vi "TAT_Manual.vi"(8 "error In":errorcluster) -> (0 "error out":errorcluster)   [LabVIEW 2017]
uses:
  <vilib>/addons/database/Connection.llb/Conn ObjectReference.ctl
  <vilib>/Utility/error.llb/DialogType.ctl
  Controls/Ass. Loop Control.ctl
  b57a9467-0384-43c0-b8a9-3ecd2744b4aa.vi
  <vilib>/Instr/_visa.llb/VISA Configure Serial Port (Instr).vi
  <vilib>/Utility/config.llb/Read Key (I32).vi
  <vilib>/addons/database/NI_Database_API.lvlib
  <vilib>/Utility/config.llb/NI_LVConfig.lvlib
  def1aff2-28af-4330-adfa-ddbbffd99805.vi
panel:
  in  "Varient Change":bool
  out "12 4":bool
  out "12 2":bool
  out "12":bool
  in  "temp":refnum<visa-resource-name>
  out "array":string[](array[string])
  out "LEAK UNIT RESULT 2":bool caption="LEAK RESULT:-"
  out "LEAK ACTUAL VALUE 2":string
  out "LEAK MAX 2":string
  out "LEAK MIN 2":string
  out "LEAK UNIT RESULT":bool caption="LEAK RESULT:-"
  out "LEAK ACTUAL VALUE":string
  out "LEAK MAX":string
  out "LEAK MIN":string
  out "PREVIOUS BARCODE":string[](array[string])
  out "scanned":string
  out "Scanned Qyt":string
  out "PROJECT :-":string
  out "PACKAGE Qty":string
  out "TORISHI CODE:-":string
  out "PART No.:-":string
  in  "Stop":bool
  out "BARCODE STATION 2":string caption="BARCODE:-"
  out "RESULT STATION 1":bool caption="FINAL RESULT:-"
  out "USER:-":string
  out "PART NAME :-":string
  in  "ASS-Alarms":bool
  out "CYCLE STATUS STATION 1":string caption="CYCLE STATUS:-"
  out "DATE/TIME":string
  # "KAPSE SONS ROBOTICS\n& AUTOMATION"
  # "PROGRAM SELECTION"
  # "PREVIOUS BARCODE"
  # "Nm"
  # "POKA-YOKE STATUS"
  # "LEAK TESTING PARAMETER"
  # "MIN"
  # "MAX"
  # "ACTUAL VALUE"
  # "RESULT"
  # "LEAK UNIT"
  # "LEAK PRESSURE"
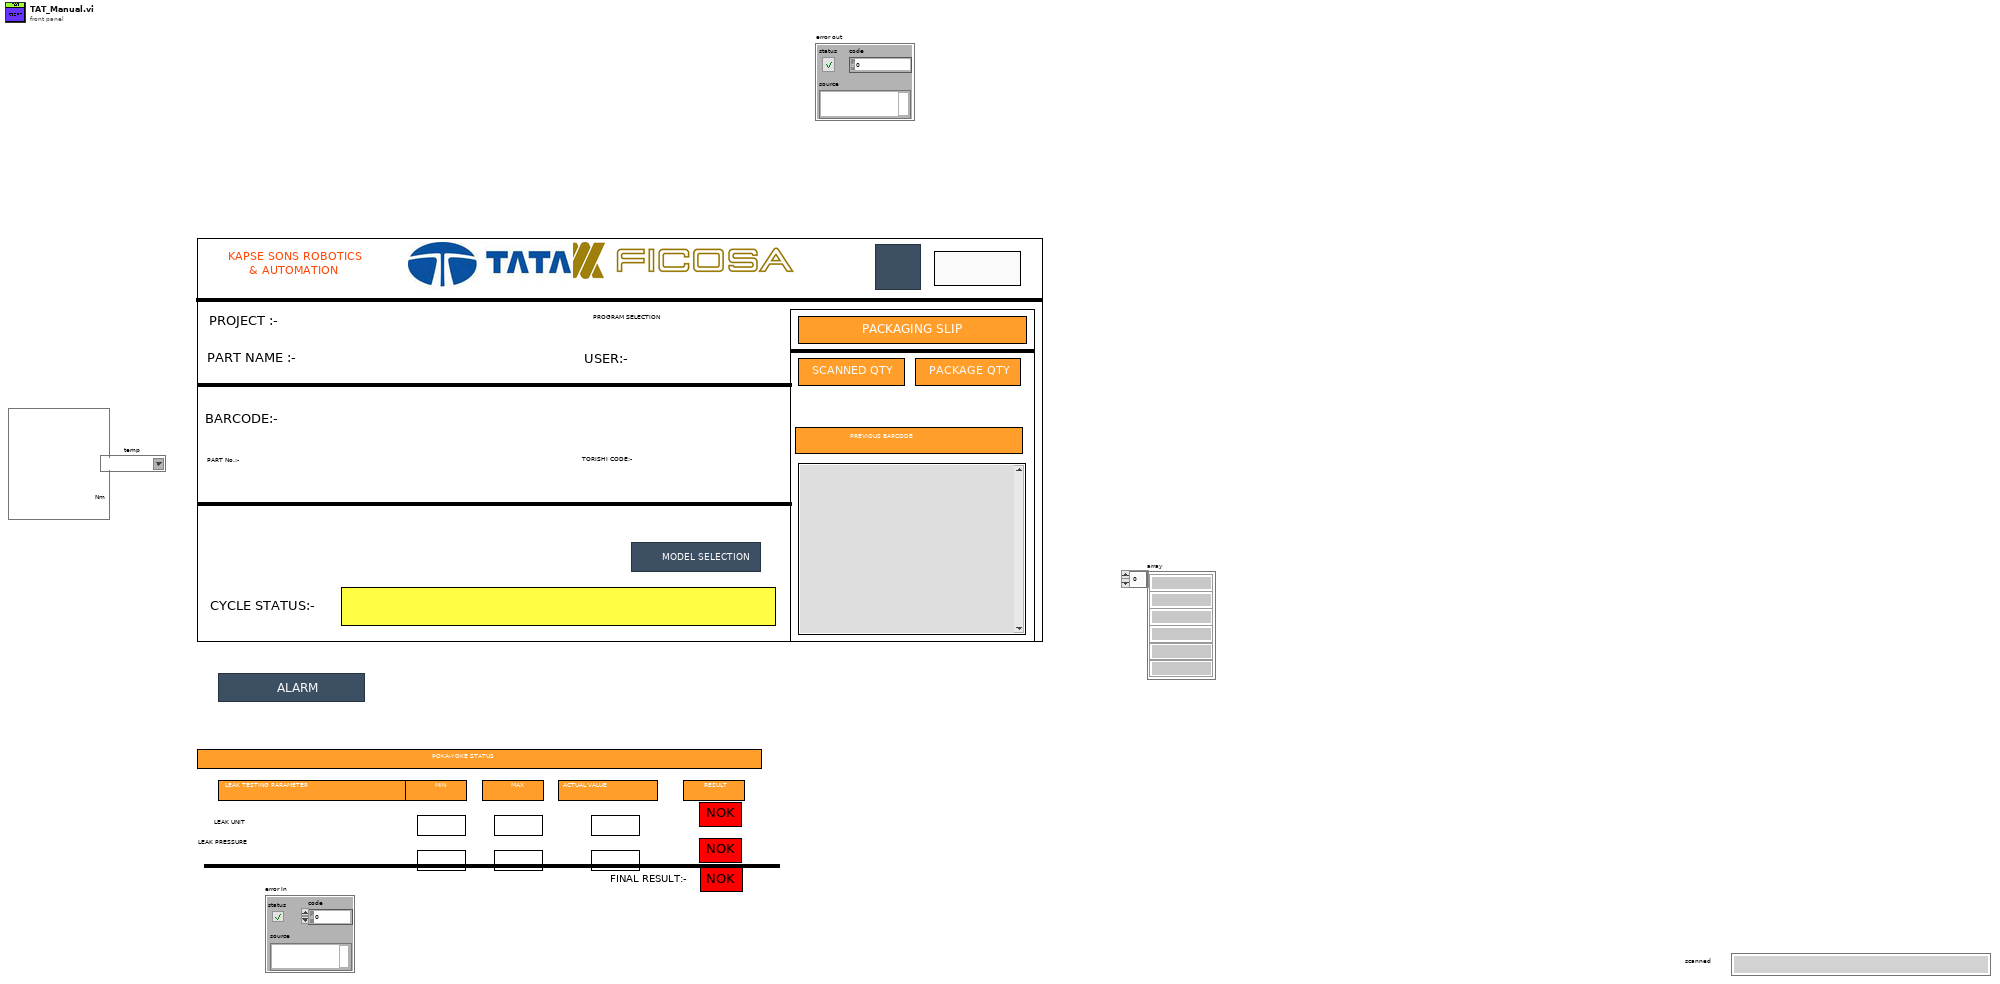
[diagram p1: front panel]
types:
  T1 = typedef "Ass. Loop Control.ctl" = enum16{"Int2", "Package_Qty_Count", "GENERATE_QR_PRNT", "Cluster_update", "Waiting_for_scan", "barcode CHECK", "Int", "SaveReport ", "Barcode Print", "Start Cycle", "Wait", "Cycle End", "Stop"}
  T2 = typedef "DialogType.ctl" = u16
  T3 = typedef "NI_Database_API.lvlib/Conn ObjectReference.ctl" = refnum<k1>
  T4 = cluster{"Varient number":u16, "Part name":string, "Barcode":string, "connection reference":T3, "Batch_Size":u16, "PART_NO":string, "TORISHI_CODE":string, "scanner com":refnum<visa-resource-name>, "Part Name List":string[], "Varient path":path, "Current Varient path":path, "Communication path":path, "PRN path":path, "printer":refnum<k5>, "Data_log_Path":path, "PREVIOUS Code":string[], "printer ip add":string}
  T5 = enum32{"invalid app kind", "Development System", "Run Time System", "Student Edition", "Embedded LabVIEW", "Evaluation", "Custom"}
  T6 = typedef "NI_LVConfig.lvlib/Config Data RefNum.ctl" = refnum<k1>
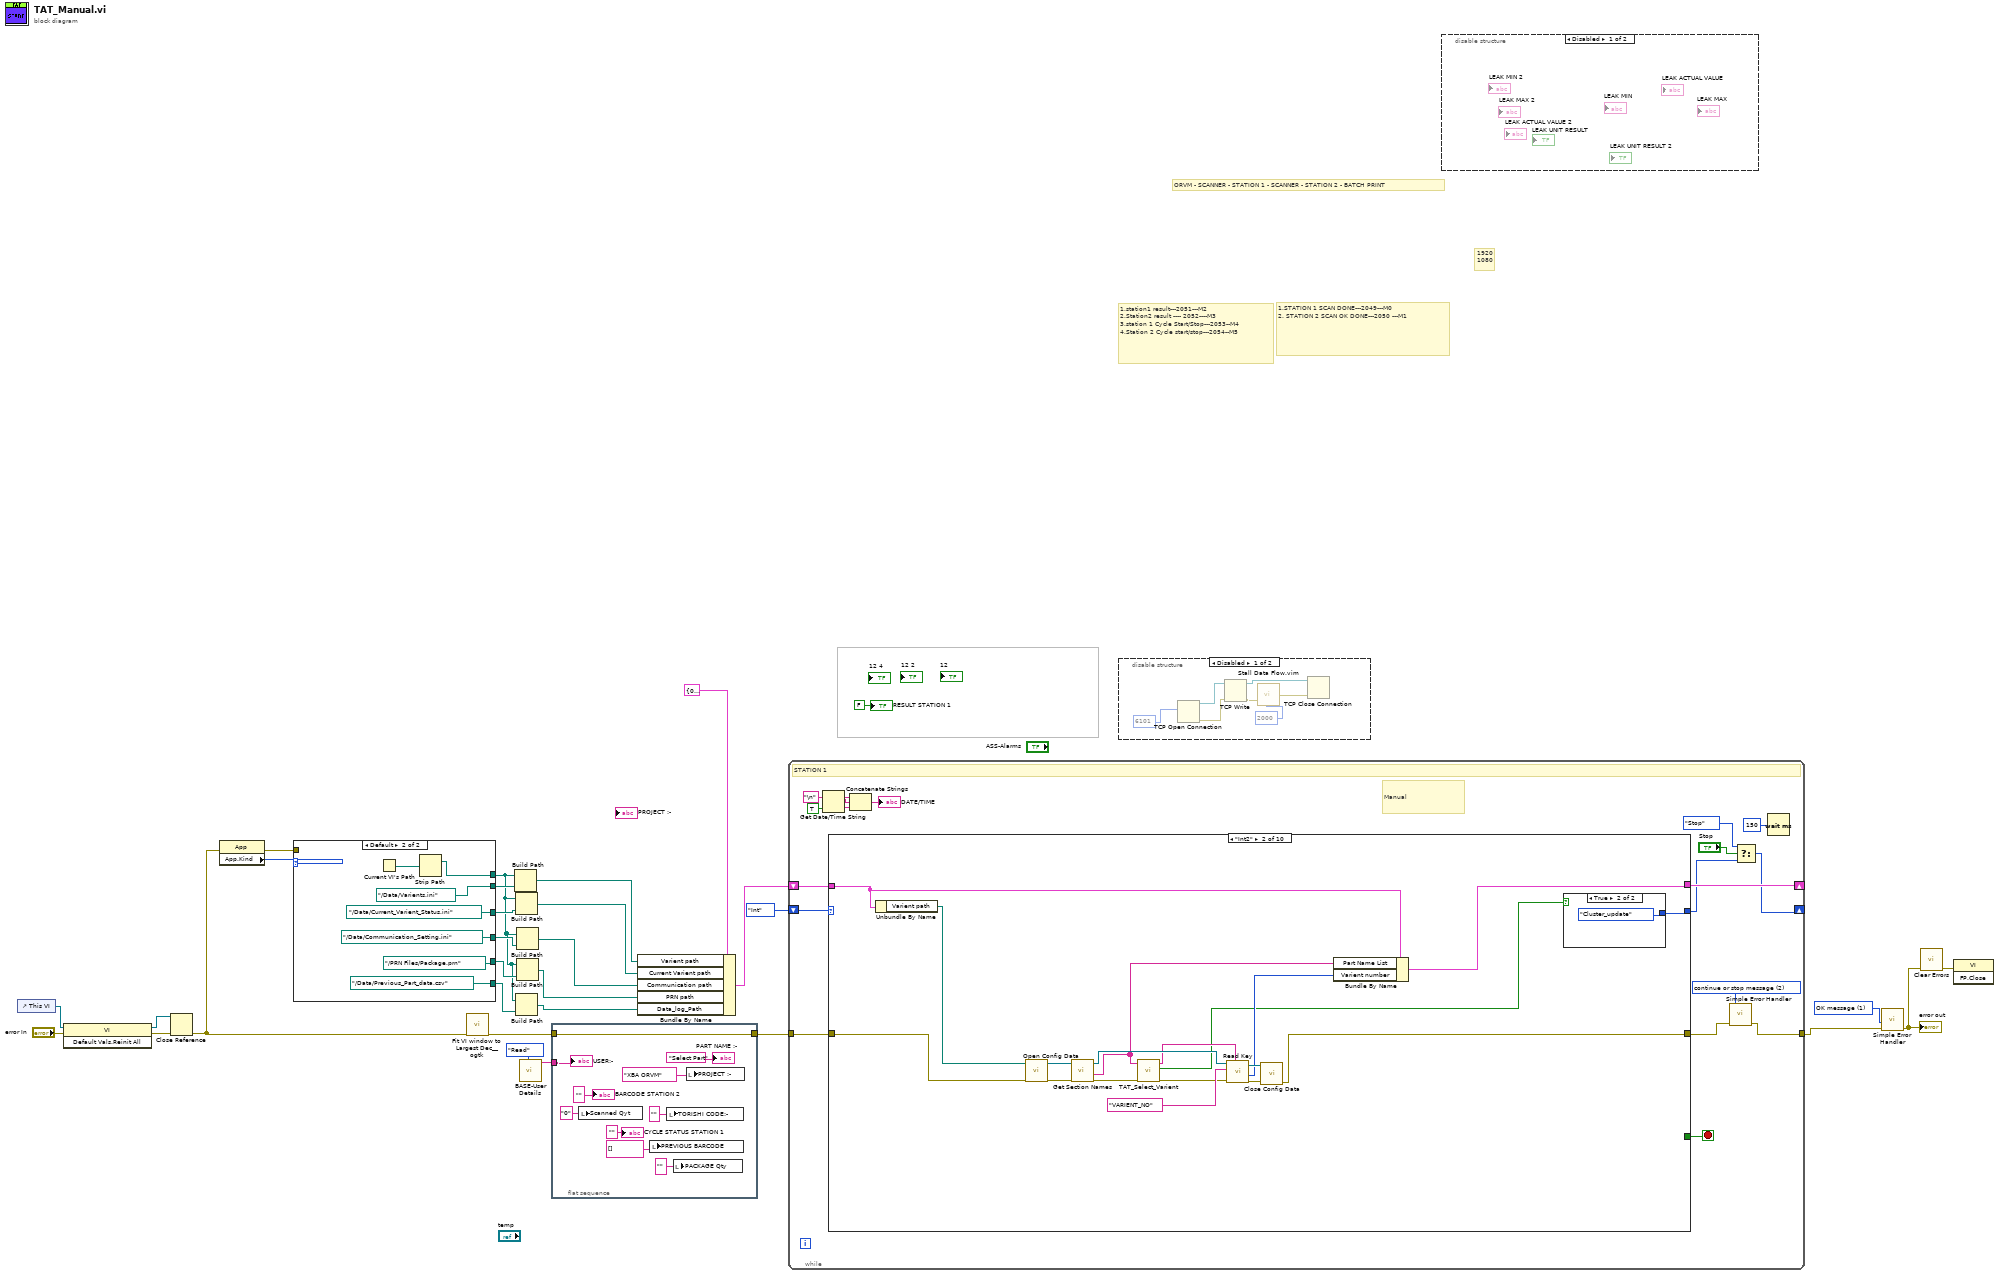
[diagram p0: block diagram]
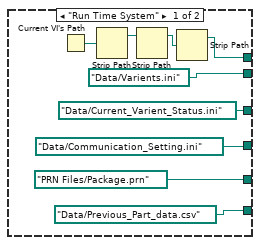
[diagram p3: hidden frame]
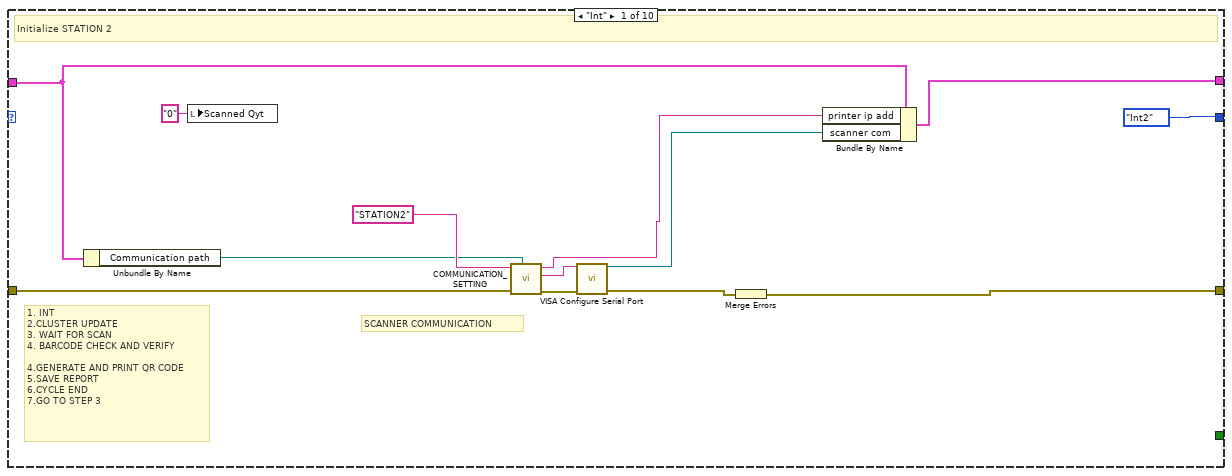
[diagram p5: hidden frame]
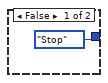
[diagram p6: hidden frame]
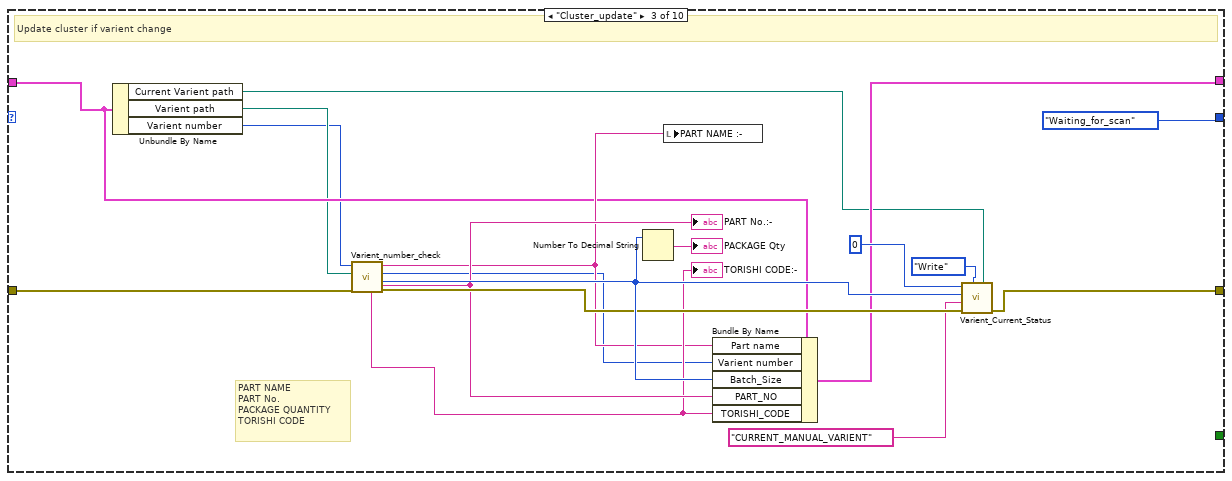
[diagram p7: hidden frame]
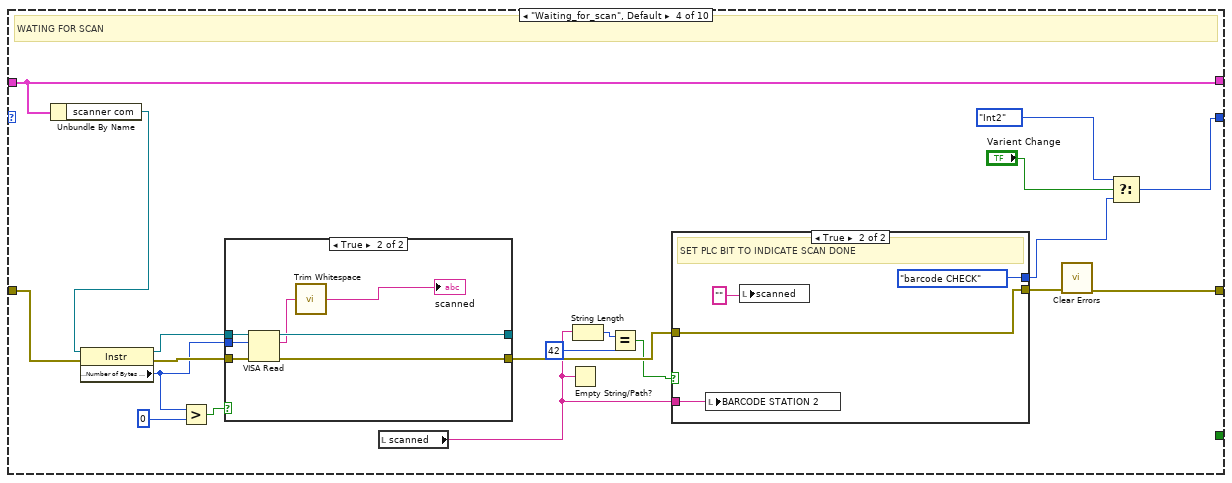
[diagram p8: hidden frame]
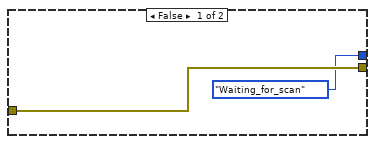
[diagram p10: hidden frame]
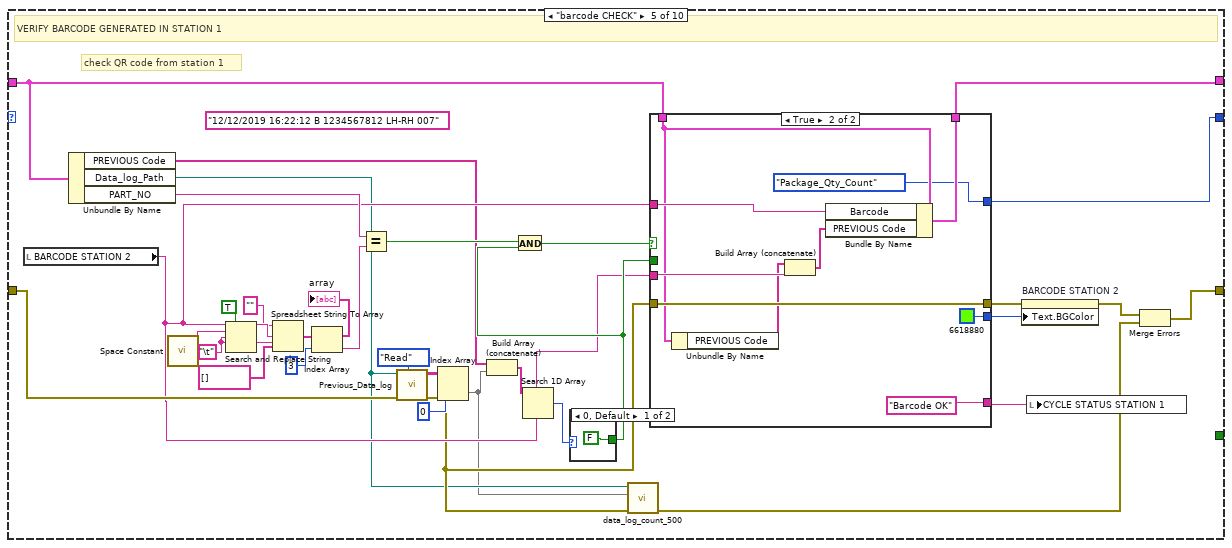
[diagram p11: hidden frame]
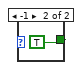
[diagram p12: hidden frame]
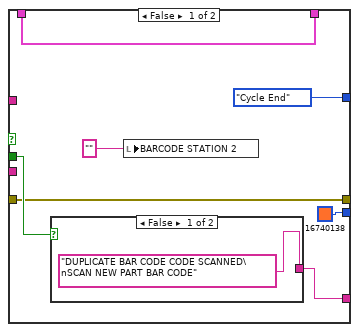
[diagram p13: hidden frame]
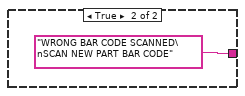
[diagram p14: hidden frame]
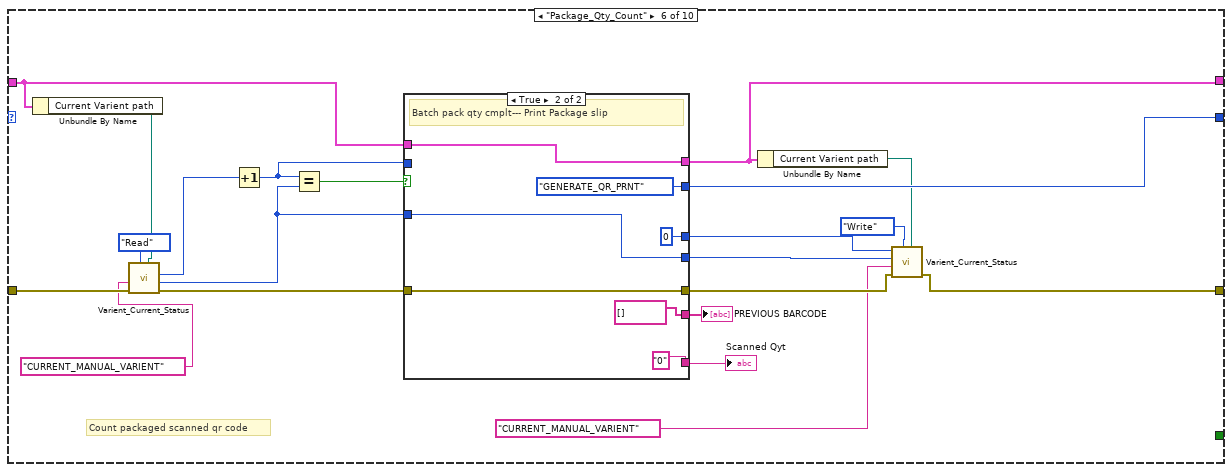
[diagram p15: hidden frame]
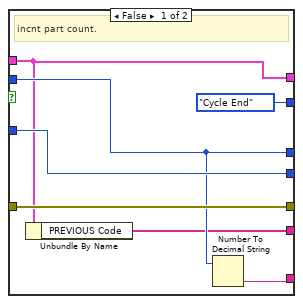
[diagram p16: hidden frame]
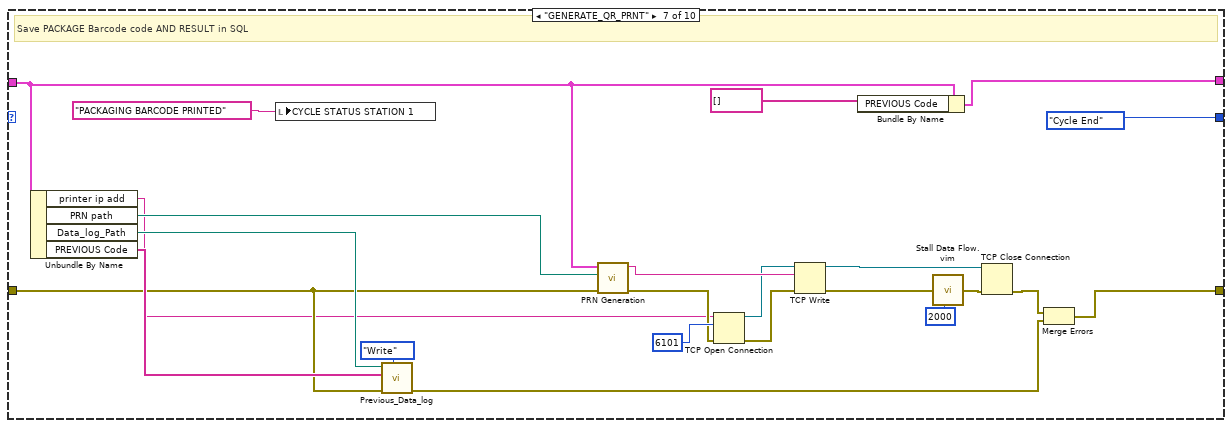
[diagram p17: hidden frame]
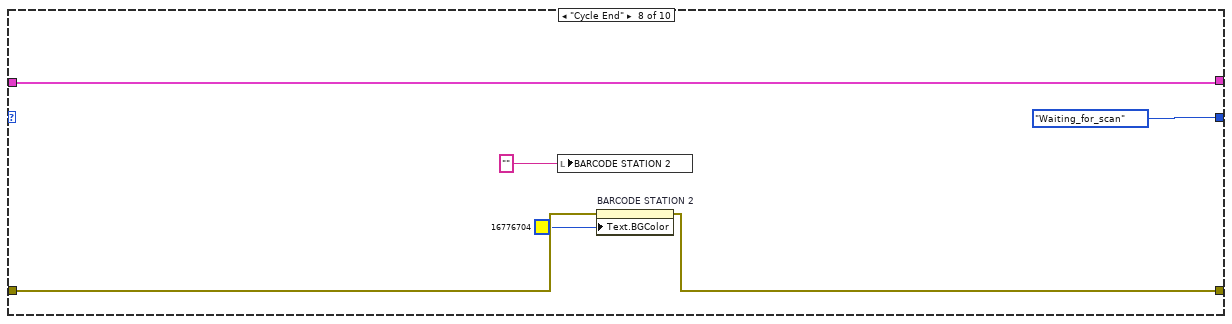
[diagram p18: hidden frame]
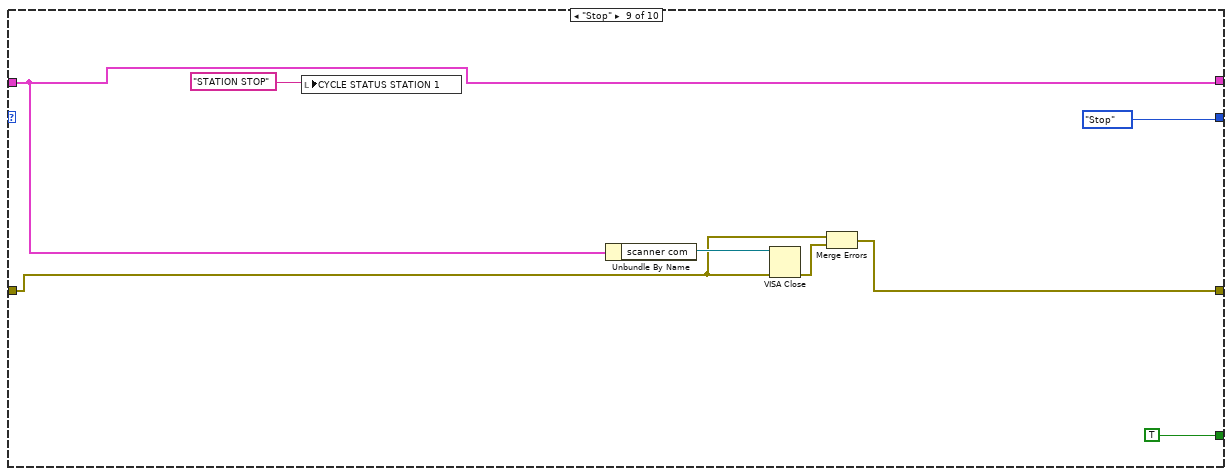
[diagram p19: hidden frame]
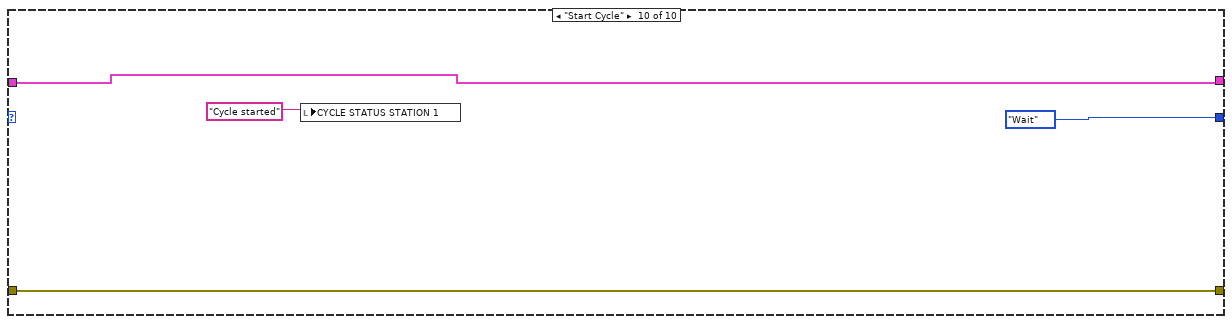
[diagram p20: hidden frame]
diagram:
  w20 = T2 1 items=["no dialog", "OK message", "continue or stop message", "OK message + warnings", "continue/stop + warnings"] ("type of dialog (OK msg:1)")
  # "1920\n1080"
  # "1.STATION 1 SCAN DONE---2049---M0\n2. STATION 2 SCAN OK DONE---2050 ---M1"
  # "1.station1 result---2051---M2\n2.Station2 result ---- 2052----M3\n3.station 1 Cycle Start/Stop---2053--M4\n4.Station 2 Cycle start/stop---2054--M5"
  # "ORVM - SCANNER - STATION 1 - SCANNER - STATION 2 - BATCH PRINT"
  n1 = control-ref of="This VI"() -> (w30:refnum<vi>)
  n2 = invoke class="VI" method="Default Vals.Reinit All"(reference=w30, error in="error In") -> (reference out=w27:refnum<vi>, error out=w28:errorcluster)  [unwired: 1 in, 1 out]
  n3 = Close Reference(reference=w27, error in (no error)=w28) -> (error out=w14:errorcluster)
  n4 = property class="App"(error in=w14) -> (error out=w4:errorcluster, "App.Kind"=w16:T5)  [unwired: 1 in, 1 out]
  n5 = case shown="Default" w16 {
    tunnel: [path "Data/Varients.ini" ("path") path "../Data/Varients.ini" ("path")] -> w15
    tunnel: [w35 w44] -> w2
    tunnel: [path "Data/Current_Varient_Status.ini" ("path") path "../Data/Current_Varient_Status.ini" ("path")] -> w9
    tunnel: [path "Data/Communication_Setting.ini" ("path") path "../Data/Communication_Setting.ini" ("path")] -> w8
    tunnel: [path "PRN Files/Package.prn" ("path") path "../PRN Files/Package.prn" ("path")] -> w6
    tunnel: w4 -> [_ _]
    tunnel: [path "Data/Previous_Part_data.csv" ("path") path "../Data/Previous_Part_data.csv" ("path")] -> w1
    frame "Run Time System" {
      n6 = Current VI's Path() -> (path=w38:path)
      n7 = Strip Path(path=w38) -> (stripped path=w37:path)  [unwired: 1 out]
      n8 = Strip Path(path=w37) -> (stripped path=w36:path)  [unwired: 1 out]
      n9 = Strip Path(path=w36) -> (stripped path=w35:path)  [unwired: 1 out]
    }
    frame Default {
      n10 = Current VI's Path() -> (path=w45:path)
      n11 = Strip Path(path=w45) -> (stripped path=w44:path)  [unwired: 1 out]
    }
  }
  n12 = call <userlib>:"Fit VI window to Largest Dec__ogtk.vi"("error in (no error)"=w14) -> ("error out"=w26:errorcluster)  [unwired: 5 in, 1 out]
  n13 = Build Path(base path=w2, name or relative path=w15) -> (appended path=w11:path)
  n14 = Build Path(base path=w2, name or relative path=w9) -> (appended path=w10:path)
  n15 = Build Path(base path=w2, name or relative path=w1) -> (appended path=w3:path)
  n16 = Build Path(base path=w2, name or relative path=w8) -> (appended path=w7:path)
  n17 = Build Path(base path=w2, name or relative path=w6) -> (appended path=w5:path)
  n18 = call "BASE-User Details.vi"("Enum"=enum16{"Read", "Write"}."Read") -> ("User Name Out"=w21:string)  [unwired: 9 in, 1 out]
  n19 = flat-sequence {
    tunnel: [w56] -> w18
    tunnel: w26 -> [w56]
    tunnel: w21 -> [w55]
    frame #0 {
      n20 = local write "Scanned Qyt"("0" ("Scanned Qyt")) -> ()
      n21 = local write "PREVIOUS BARCODE"(string[] [] ("PREVIOUS BARCODE")) -> ()
      n22 = local write "TORISHI CODE:-"("") -> ()
      n23 = local write "PACKAGE Qty"("") -> ()
      n24 = local write "PROJECT :-"("XBA ORVM" ("PROJECT")) -> ()
      "USER:-" <- w55
      "PART NAME :-" <- "Select Part"
      "BARCODE STATION 2" <- ""
      "CYCLE STATUS STATION 1" <- ""
    }
  }
  n25 = Bundle By Name(cluster=T4 {"Varient number"=0, "Part name"="", "Barcode"="", "connection reference"=refnum, "Batch_Size"=0, "PART_NO"="", "TORISHI_CODE"="", "scanner com"="", "Part Name List"=[], "Varient path"=path "", "Current Varient path"=path "", "Communication path"=path "", "PRN path"=path "", "printer"=refnum, "Data_log_Path"=path "", "PREVIOUS Code"=[], "printer ip add"=""}, "Varient path"=w11, "Current Varient path"=w10, "Communication path"=w7, "PRN path"=w5, "Data_log_Path"=w3) -> (w12:T4)
  n26 = while {
    shift-right: [w63] -> _
    shift-left: Ass._Loop_Control."Int" ("Enum") -> [w68]
    tunnel: w18 -> [w67]
    shift-right: [w65] -> _
    shift-left: w12 -> [w66]
    tunnel: [w58] -> w17
    stop <- w57 stop-if-true
    w60 = T2 2 items=["no dialog", "OK message", "continue or stop message", "OK message + warnings", "continue/stop + warnings"] ("type of dialog (OK msg:1)")
    # "Manual"
    # "STATION 1"
    n27 = Get Date/Time String(want seconds? (F)=TRUE) -> (date string=w72:string, time string=w71:string)  [unwired: 2 in]
    n28 = case shown="\"Int2\"" w68 {
      tunnel: [Ass._Loop_Control."Int2" ("Enum") w93 Ass._Loop_Control."Waiting_for_scan" ("Enum") w126 w168 w223 Ass._Loop_Control."Cycle End" ("Enum") Ass._Loop_Control."Waiting_for_scan" ("Enum") Ass._Loop_Control."Stop" ("Enum") Ass._Loop_Control."Wait" ("Enum")] -> w62
      tunnel: [w77 w96 w113 w138 w190 w214 w261 w276 w281 w286] -> w65
      tunnel: [w78 w88 w116 w144 w166 w228 w260 w274 w282 w287] -> w59
      tunnel: w67 -> [w84 w89 w115 w139 w176 w234 w259 w275 w279 w287]
      tunnel: w66 -> [w83 w91 w114 w138 w191 w215 w257 w276 w281 w286]
      tunnel: [_ _ _ _ _ _ _ _ TRUE _] -> w57
      frame "Int" {
        # "1. INT\n2.CLUSTER UPDATE\n3. WAIT FOR SCAN\n4. BARCODE CHECK AND VERIFY\n\n4.GENERATE AND PRINT QR CODE\n5.SAVE REPORT\n6.CYCLE END\n7.GO TO STEP 3"
        # "SCANNER COMMUNICATION"
        # "Initialize STATION 2"
        n29 = Unbundle By Name(w83) -> ("Communication path"=w82:path)
        n30 = local write "Scanned Qyt"("0" ("Scanned Qyt")) -> ()
        n31 = call "COMMUNICATION_SETTING.vi"("communication path"=w82, "error in"=w84, "STATION"="STATION2") -> ("error out"=w87:errorcluster, "SCAN_COM"=w85:string, "PRINT_COM"=w75:string)  [unwired: 6 in]
        n32 = call-poly "VISA Configure Serial Port"("VISA resource name"=w85, "error in (no error)"=w87) -> ("VISA resource name out"=w80:refnum<visa-resource-name>, "error out"=w79:errorcluster)  [unwired: 12 in]
        n33 = Merge Errors(w79) -> (w78:errorcluster)
        n34 = Bundle By Name(cluster=w83, "printer ip add"=w75, "scanner com"=w80) -> (w77:T4)
      }
      frame "Int2" {
        n35 = Unbundle By Name(w91) -> ("Varient path"=w90:path)
        n36 = call <vilib>:"Open Config Data.vi"("error in (no error)"=w89, "configuration file path"=w90) -> ("error out"=w104:errorcluster, "refnum"=w105:T6)  [unwired: 7 in, 1 out]
        n37 = call <vilib>:"Get Section Names.vi"("error in (no error)"=w104, "refnum"=w105) -> ("error out"=w103:errorcluster, "section names"=w95:string[], "refnum out"=w98:T6)  [unwired: 7 in]
        n38 = call "TAT_Select_Varient.vi"("Part List"=w95, "Error In"=w103) -> ("User Name Out"=w97:string, "Cancle"=w92:bool, "error out"=w101:errorcluster)  [unwired: 5 in, 1 out]
        n39 = call-poly <vilib>:"Read Key.vi"("section"=w97, "error in (no error)"=w101, "key"="VARIENT_NO" ("name or relative path"), "refnum"=w98) -> ("error out"=w100:errorcluster, "value"=w94:i32, "refnum out"=w99:T6)  [unwired: 4 in, 1 out]
        n40 = call <vilib>:"Close Config Data.vi"("error in (no error)"=w100, "refnum"=w99) -> ("error out"=w88:errorcluster)  [unwired: 8 in, 1 out]
        n41 = Bundle By Name(cluster=w91, "Part Name List"=w95, "Varient number"=w94) -> (w96:T4)
        n42 = case shown="True" w92 {
          tunnel: [Ass._Loop_Control."Stop" ("Enum") Ass._Loop_Control."Cluster_update" ("Enum")] -> w93
          frame False {
          }
          frame True {
          }
        }
      }
      frame "Cluster_update" {
        # "PART NAME\nPART No.\nPACKAGE QUANTITY\nTORISHI CODE"
        # "Update cluster if varient change"
        n43 = Unbundle By Name(w114) -> ("Current Varient path"=w109:path, "Varient path"=w110:path, "Varient number"=w108:u16)
        n44 = call "Varient_number_check.vi"("error in"=w115, "Varient path"=w110, "Varient No."=w108) -> ("error out"=w124:errorcluster, "Batch Size"=w125:i32, "Varient Number"=w119:i32, "Part Name"=w120:string, "PART_NO"=w123:string, "TORISHI_CODE"=w122:string)  [unwired: 2 in, 1 out]
        "PART No.:-" <- w123
        "TORISHI CODE:-" <- w122
        n45 = Number To Decimal String(number=w125) -> (decimal integer string=→"PACKAGE Qty":string)  [unwired: 1 in]
        n46 = local write "PART NAME :-"(w120) -> ()
        n47 = Bundle By Name(cluster=w114, "Part name"=w120, "Varient number"=w119, "Batch_Size"=w125, "PART_NO"=w123, "TORISHI_CODE"=w122) -> (w113:T4)
        n48 = call "Varient_Current_Status.vi"("Currenrt Varient path"=w109, "Enum"=enum16{"Write", "Read"}."Write", "error in"=w124, "AUTO/MANUAL"="CURRENT_MANUAL_VARIENT", "Batch Size"=w125, "Varient count"=0) -> ("error out"=w116:errorcluster)  [unwired: 3 in, 2 out]
      }
      frame "Waiting_for_scan", Default {
        # "WATING FOR SCAN"
        n49 = Unbundle By Name(w138) -> ("scanner com"=w137:refnum<visa-resource-name>)
        n50 = property class="Instr"(reference=w137, error in=w139) -> (reference out=w143:refnum<visa-resource-name>, error out=w142:errorcluster, "Serial Settings:Number of Bytes at Serial Port"=w136:u32)
        n51 = Greater?(x=w136, y=u32 0) -> (0:w135:bool)
        n52 = case shown="True" w135 {
          tunnel: w143 -> [w146 w153]
          tunnel: w142 -> [w145 w152]
          tunnel: w136 -> [_ w151]
          tunnel: [w146 w150] -> _
          tunnel: [w145 w147] -> w141
          frame False {
          }
          frame True {
            n53 = VISA Read(VISA resource name=w153, byte count=w151, error in (no error)=w152) -> (VISA resource name out=w150:refnum<visa-resource-name>, read buffer=w148:string, error out=w147:errorcluster)  [unwired: 1 out]
            n54 = call <vilib>:"Trim Whitespace.vi"("string"=w148) -> ("trimmed string"=→"scanned":string)  [unwired: 1 in]
          }
        }
        n55 = local read "scanned"() -> (w133:string)
        n56 = Empty String/Path?(string/path=w133) -> ()  [unwired: 1 out]
        n57 = String Length(string=w133) -> (length=w132:i32)
        n58 = Equal?(x=w132, y=42) -> (x = y?=w130:bool)
        n59 = case shown="True" w130 {
          tunnel: w141 -> [w155 w159]
          tunnel: [w155 w159] -> w140
          tunnel: w133 -> [_ w158]
          tunnel: [Ass._Loop_Control."Waiting_for_scan" ("Enum") Ass._Loop_Control."barcode CHECK" ("Enum")] -> w127
          frame False {
          }
          frame True {
            # "SET PLC BIT TO INDICATE SCAN DONE"
            n60 = local write "BARCODE STATION 2"(w158) -> ()
            n61 = local write "scanned"("") -> ()
          }
        }
        n62 = call <vilib>:"Clear Errors.vi"("error in (no error)"=w140) -> ("error out"=w144:errorcluster)  [unwired: 5 in, 1 out]
        n63 = Select(t=Ass._Loop_Control."Int2" ("Enum"), s="Varient Change", f=w127) -> (s? t:f=w126:T1)
      }
      frame "barcode CHECK" {
        w186 = "\t"
        (unwired) "12/12/2019 16:22:12 B 1234567812 LH-RH 007" ("string")
        # "check QR code from station 1"
        # "VERIFY BARCODE GENERATED IN STATION 1"
        n64 = local read "BARCODE STATION 2"() -> (w170:string)
        n65 = Unbundle By Name(w191) -> ("PREVIOUS Code"=w162:string[], "Data_log_Path"=w163:path, "PART_NO"=w182:string)
        n66 = call <vilib>:"Space Constant.vi"() -> ("String"=w189:string)
        n67 = Search and Replace String(replace all?=TRUE ("replace all? (F)"), input string=w170, search string=w189, replace string=w186) -> (result string=w187:string)  [unwired: 4 in, 3 out]
        n68 = Spreadsheet String To Array(delimiter (Tab)=w186, format string="", spreadsheet string=w187, array type (2D Dbl)=string[] []) -> (array=w178:string[])
        "array" <- w178
        n69 = Index Array(array=w178, index=3) -> (element=w181:string)
        n70 = Equal?(x=w182, y=w181) -> (x = y?=w180:bool)
        n71 = call "Previous_Data_log.vi"(7:enum16{"Write", "Read"}."Read", "error in (no error)"=w176, "file path (dialog if empty)"=w163) -> ("error out"=w164:errorcluster, "all rows"=w174:string[][])  [unwired: 7 in]
        n72 = Index Array(array=w174, index (col)=0 ("disabled index (col)")) -> (element=w160:string[])  [unwired: 1 in]
        n73 = Build Array (concatenate)(w162, w160) -> (w161:string[])
        n74 = Search 1D Array(1D array=w161, element=w170) -> (index of element=w172:i32)  [unwired: 1 in]
        n75 = case shown="0, Default" w172 {
          tunnel: [FALSE TRUE] -> w171
          frame 0, Default {
          }
          frame -1 {
          }
        }
        n76 = And(x=w180, y=w171) -> (x .and. y?=w179:bool)
        n77 = call "data_log_count_500.vi"("error in (no error)"=w164, "All data"=w160, "file path (dialog if empty)"=w163) -> ("error out"=w165:errorcluster)  [unwired: 8 in]
        n78 = case shown="True" w179 {
          tunnel: [w201 "Barcode OK" ("Cycle Status")] -> w192
          tunnel: w191 -> [w200 w207]
          tunnel: [w200 w212] -> w190
          tunnel: w170 -> [_ w211]
          tunnel: w171 -> [w199 _]
          tunnel: w170 -> [_ w210]
          tunnel: [u32 16740138 u32 6618880] -> w177
          tunnel: w164 -> [w197 w208]
          tunnel: [w197 w208] -> w169
          tunnel: [Ass._Loop_Control."Cycle End" ("Enum") Ass._Loop_Control."Package_Qty_Count" ("Enum")] -> w168
          frame False {
            n79 = case shown="False" w199 {
              tunnel: ["DUPLICATE BAR CODE CODE SCANNED\nSCAN NEW PART BAR CODE" ("Cycle Status") "WRONG BAR CODE SCANNED\nSCAN NEW PART BAR CODE" ("Cycle Status")] -> w201
              frame False {
              }
              frame True {
              }
            }
            n80 = local write "BARCODE STATION 2"("") -> ()
          }
          frame True {
            n81 = Unbundle By Name(w207) -> ("PREVIOUS Code"=w206:string[])
            n82 = Build Array (concatenate)(w206, w210) -> (w205:string[])
            n83 = Bundle By Name(cluster=w207, "Barcode"=w211, "PREVIOUS Code"=w205) -> (w212:T4)
          }
        }
        n84 = property on="BARCODE STATION 2" class="Str"(error in=w169, "Text.BGColor"=w177) -> (error out=w167:errorcluster)  [unwired: 1 in, 1 out]
        n85 = local write "CYCLE STATUS STATION 1"(w192) -> ()
        n86 = Merge Errors(w167, w165) -> (w166:errorcluster)
      }
      frame "Package_Qty_Count" {
        # "Count packaged scanned qr code"
        n87 = Unbundle By Name(w215) -> ("Current Varient path"=w219:path)
        n88 = call "Varient_Current_Status.vi"("Currenrt Varient path"=w219, "Enum"=enum16{"Write", "Read"}."Read", "error in"=w234, "AUTO/MANUAL"="CURRENT_MANUAL_VARIENT") -> ("error out"=w232:errorcluster, "Batch Size"=w226:i32, "Varient Count"=w231:i32)  [unwired: 5 in]
        n89 = Increment(x=w231) -> (x+1=w218:i32)
        n90 = Equal?(x=w218, y=w226) -> (x = y?=w230:bool)
        n91 = case shown="True" w230 {
          tunnel: [w241 w248] -> w227
          tunnel: w232 -> [w241 w248]
          tunnel: w218 -> [w237 _]
          tunnel: w226 -> [w240 w247]
          tunnel: [w240 w247] -> w225
          tunnel: [w237 0] -> w224
          tunnel: [Ass._Loop_Control."Cycle End" ("Enum") Ass._Loop_Control."GENERATE_QR_PRNT" ("Enum")] -> w223
          tunnel: [w236 string[] [] ("PREVIOUS BARCODE")] -> w217
          tunnel: [w238 "0"] -> w216
          tunnel: w215 -> [w235 w242]
          tunnel: [w235 w242] -> w214
          frame False {
            # "incnt part count."
            n92 = Unbundle By Name(w235) -> ("PREVIOUS Code"=w236:string[])
            n93 = Number To Decimal String(number=w237) -> (decimal integer string=w238:string)  [unwired: 1 in]
          }
          frame True {
            # "Batch pack qty cmplt--- Print Package slip"
          }
        }
        "PREVIOUS BARCODE" <- w217
        "Scanned Qyt" <- w216
        n94 = Unbundle By Name(w214) -> ("Current Varient path"=w220:path)
        n95 = call "Varient_Current_Status.vi"("Currenrt Varient path"=w220, "Enum"=enum16{"Write", "Read"}."Write", "error in"=w227, "AUTO/MANUAL"="CURRENT_MANUAL_VARIENT", "Batch Size"=w225, "Varient count"=w224) -> ("error out"=w228:errorcluster)  [unwired: 3 in, 2 out]
      }
      frame "GENERATE_QR_PRNT" {
        # "Save PACKAGE Barcode code AND RESULT in SQL"
        n96 = Unbundle By Name(w257) -> ("printer ip add"=w252:string, "PRN path"=w266:path, "Data_log_Path"=w263:path, "PREVIOUS Code"=w262:string[])
        n97 = local write "CYCLE STATUS STATION 1"("PACKAGING BARCODE PRINTED" ("Cycle Status")) -> ()
        n98 = call "Previous_Data_log.vi"(7:enum16{"Write", "Read"}."Write", "error in (no error)"=w259, "Data IN"=w262, "file path (dialog if empty)"=w263) -> ("error out"=w258:errorcluster)  [unwired: 6 in, 1 out]
        n99 = call "PRN Generation.vi"("error in (no error)"=w259, "PRN path"=w266, "Cluster"=w257) -> ("error out"=w255:errorcluster, "PRN to Print"=w269:string)  [unwired: 7 in]
        n100 = TCP Open Connection(address=w252, remote port or service name=u16 6101, error in (no error)=w255) -> (connection ID=w253:refnum<k5>, error out=w254:errorcluster)  [unwired: 2 in]
        n101 = TCP Write(connection ID=w253, data in=w269, error in (no error)=w254) -> (connection ID out=w249:refnum<k5>, error out=w268:errorcluster)  [unwired: 1 in, 1 out]
        n102 = Bundle By Name(cluster=w257, "PREVIOUS Code"=string[] []) -> (w261:T4)
        n103 = call "Stall Data Flow.vim"("value in"=w268, "milliseconds to wait"=u32 2000) -> ("value out"=w251:errorcluster)  [unwired: 1 out]
        n104 = TCP Close Connection(connection ID=w249, error in (no error)=w251) -> (error out=w250:errorcluster)  [unwired: 1 in, 1 out]
        n105 = Merge Errors(w250, w258) -> (w260:errorcluster)
      }
      frame "Cycle End" {
        n106 = local write "BARCODE STATION 2"("" ("BARCODE STATION 2")) -> ()
        n107 = property on="BARCODE STATION 2" class="Str"(error in=w275, "Text.BGColor"=u32 16776704) -> (error out=w274:errorcluster)  [unwired: 1 in, 1 out]
      }
      frame "Stop" {
        n108 = local write "CYCLE STATUS STATION 1"("STATION STOP" ("Cycle Status")) -> ()
        n109 = Unbundle By Name(w281) -> ("scanner com"=w280:refnum<visa-resource-name>)
        n110 = VISA Close(VISA resource name=w280, error in (no error)=w279) -> (error out=w283:errorcluster)
        n111 = Merge Errors(w279, w283) -> (w282:errorcluster)
      }
      frame "Start Cycle" {
        n112 = local write "CYCLE STATUS STATION 1"("Cycle started" ("Cycle Status")) -> ()
      }
    }
    n113 = Concatenate Strings(w72, "\n", w71) -> (→"DATE/TIME":string)
    n114 = call <vilib>:"Simple Error Handler.vi"("type of dialog (OK msg:1)"=w60, "error in (no error)"=w59) -> ("error out"=w58:errorcluster)  [unwired: 3 in, 4 out]
    n115 = Select(t=Ass._Loop_Control."Stop" ("Enum"), s="Stop", f=w62) -> (s? t:f=w63:T1)
    n116 = Wait (ms)(milliseconds to wait=u32 150) -> ()  [unwired: 1 out]
  }
  n117 = disable-structure shown="Disabled" {
    frame Disabled {
      n118 = TCP Open Connection(remote port or service name=u16 6101) -> (connection ID=w294:refnum<k5>, error out=w293:errorcluster)  [unwired: 4 in]
      n119 = TCP Write(connection ID=w294, error in (no error)=w293) -> (connection ID out=w296:refnum<k5>, error out=w292:errorcluster)  [unwired: 2 in, 1 out]
      n120 = call "Stall Data Flow.vim"("value in"=w292, "milliseconds to wait"=u32 2000) -> ("value out"=w295:errorcluster)  [unwired: 1 out]
      n121 = TCP Close Connection(connection ID=w296, error in (no error)=w295) -> ()  [unwired: 1 in, 2 out]
    }
    frame Enabled {
    }
  }
  n122 = disable-structure shown="Disabled" {
    frame Disabled {
    }
    frame Enabled {
    }
  }
  n123 = call <vilib>:"Simple Error Handler.vi"("type of dialog (OK msg:1)"=w20, "error in (no error)"=w17) -> ("error out"=w24:errorcluster)  [unwired: 3 in, 4 out]
  "error out" <- w24
  n124 = call <vilib>:"Clear Errors.vi"("error in (no error)"=w24) -> ("error out"=w23:errorcluster)  [unwired: 5 in, 1 out]
  n125 = invoke class="VI" method="FP.Close"(error in=w23) -> ()  [unwired: 2 in, 3 out]
  "RESULT STATION 1" <- FALSE ("want seconds? (F)")
